vi "GetFusedHeading.vi"(11 "navX Device TypeDef":T1={"navX Interface Protocol"=enum."SPI", "navX Interface Protocol TypeDefs"={"SPIDevRef"={"DevStatus"={"status"=FALSE, "code"=0, "source"=""}, "Handle"=0, "SPI Bus"=enum."SPI On-Board, CS0"}, "I2CDevRef"={"DevStatus"={"status"=FALSE, "code"=0, "source"=""}, "Device Address"=0, "Handle"=0, "I2C Bus"=enum."Invalid"}}, "navX System Information"={"Board Information"={"WhoAmI (50 | 0x32)"=0, "Board Revision"=0, "Firmware Major Version"=0, "Firmware Minor Version"=0, "NAVX_BOARD_CAPABILITY"={"OMNIMOUNT"=FALSE, "YAW_RESET"=FALSE, "VEL_AND_DISP"=FALSE}, "NAVX_BOARD_YAW_AXIS"={"BOARD_YAW_AXIS_UP"=FALSE, "BOARD_YAW_AXIS"=0}}, "Status"={"Update Rate Hz"=0, "Accelerometer Full-Scale Range"=0, "Gyro Full-Scale Range"=0, "NAVX_OP_STATUS"=0, "NAVX_CAL_STATUS"=0, "NAVX_SELFTEST_STATUS"=0, "NAVX_SENSOR_STATUS"={"MOVING"=FALSE, "YAW_STABLE"=FALSE, "MAG_DISTURBANCE"=FALSE, "ALTITUDE_VALID"=FALSE, "SEALEVEL_PRESS_SET"=FALSE, "FUSED_HEADING_VALID"=FALSE}}, "Offsets"={"Yaw"=0.0, "Quat W"=0.0, "Quat X"=0.0, "Quat Y"=0.0, "Quat Z"=0.0}, "LastSampleTimestamp"=0.0, "LastSampleValid"=FALSE}, "navX Common Information"={"Update Rate (4Hz-60Hz)"=50, "refnum name"="", "error"={"status"=FALSE, "code"=0, "source"=""}, "LastSampleFPGATimestamp"=0.0}} {"navX Common Information"."Update Rate (4Hz-60Hz)" min=4 max=60 step=1; "navX System Information"."Status"."NAVX_OP_STATUS" items=["INITIALIZING", "SELFTEST_IN_PROGRESS", "ERROR", "IMU_AUTOCAL_IN_PROGRESS", "NORMAL"]; "navX System Information"."Status"."NAVX_CAL_STATUS" items=["IMU_CAL_STATE_MASK"=3, "IMU_CAL_INPROGRESS"=0, "IMU_CAL_ACCUMULATE"=1, "IMU_CAL_COMPLETE"=2, "MAG_CAL_COMPLETE"=4, "BARO_CAL_COMPLETE"=8]; "navX Interface Protocol TypeDefs"."I2CDevRef"."Device Address" format="%.0x"}) -> (1 "Valid?":bool, 2 "Fused Heading":dbl, 3 "navX Device TypeDef":T1={"navX Interface Protocol"=enum."SPI", "navX Interface Protocol TypeDefs"={"SPIDevRef"={"DevStatus"={"status"=FALSE, "code"=0, "source"=""}, "Handle"=0, "SPI Bus"=enum."SPI On-Board, CS0"}, "I2CDevRef"={"DevStatus"={"status"=FALSE, "code"=0, "source"=""}, "Device Address"=0, "Handle"=0, "I2C Bus"=enum."Invalid"}}, "navX System Information"={"Board Information"={"WhoAmI (50 | 0x32)"=0, "Board Revision"=0, "Firmware Major Version"=0, "Firmware Minor Version"=0, "NAVX_BOARD_CAPABILITY"={"OMNIMOUNT"=FALSE, "YAW_RESET"=FALSE, "VEL_AND_DISP"=FALSE}, "NAVX_BOARD_YAW_AXIS"={"BOARD_YAW_AXIS_UP"=FALSE, "BOARD_YAW_AXIS"=0}}, "Status"={"Update Rate Hz"=0, "Accelerometer Full-Scale Range"=0, "Gyro Full-Scale Range"=0, "NAVX_OP_STATUS"=0, "NAVX_CAL_STATUS"=0, "NAVX_SELFTEST_STATUS"=0, "NAVX_SENSOR_STATUS"={"MOVING"=FALSE, "YAW_STABLE"=FALSE, "MAG_DISTURBANCE"=FALSE, "ALTITUDE_VALID"=FALSE, "SEALEVEL_PRESS_SET"=FALSE, "FUSED_HEADING_VALID"=FALSE}}, "Offsets"={"Yaw"=0.0, "Quat W"=0.0, "Quat X"=0.0, "Quat Y"=0.0, "Quat Z"=0.0}, "LastSampleTimestamp"=0.0, "LastSampleValid"=FALSE}, "navX Common Information"={"Update Rate (4Hz-60Hz)"=50, "refnum name"="", "error"={"status"=FALSE, "code"=0, "source"=""}, "LastSampleFPGATimestamp"=0.0}} {"navX Common Information"."Update Rate (4Hz-60Hz)" min=4 max=60 step=1; "navX System Information"."Status"."NAVX_OP_STATUS" items=["INITIALIZING", "SELFTEST_IN_PROGRESS", "ERROR", "IMU_AUTOCAL_IN_PROGRESS", "NORMAL"]; "navX System Information"."Status"."NAVX_CAL_STATUS" items=["IMU_CAL_STATE_MASK"=3, "IMU_CAL_INPROGRESS"=0, "IMU_CAL_ACCUMULATE"=1, "IMU_CAL_COMPLETE"=2, "MAG_CAL_COMPLETE"=4, "BARO_CAL_COMPLETE"=8]; "navX Interface Protocol TypeDefs"."I2CDevRef"."Device Address" format="%.0x"})   [LabVIEW 2015, in "navX-MXP IMU.lvlib"]
doc: "This VI gets Fused Heading data from a navX MXP unit."
uses:
  navX-MXP IMU.lvlib
  TypeDefs/navX Device TypeDef.ctl
  TypeDefs/Value TypeDefs/navX Interface Protocol.ctl
  <vilib>/Rock Robotics/WPI/SPI/WPI_SPIDevRef.ctl
  <vilib>/Rock Robotics/SystemInterfaces/spilib/spi_bus.ctl
  <vilib>/Rock Robotics/WPI/I2C/WPI_I2CDevRef.ctl
  <vilib>/Rock Robotics/SystemInterfaces/i2clib/i2c_bus.ctl
  TypeDefs/Data TypeDefs/navX Board Information.ctl
  TypeDefs/Value TypeDefs/navX NAVX_BOARD_CAPABILITY.ctl
  TypeDefs/Value TypeDefs/navX NAVX_BOARD_YAW_AXIS.ctl
  TypeDefs/Data TypeDefs/navX Status Data.ctl
  TypeDefs/Value TypeDefs/navX NAVX_OP_STATUS.ctl
  TypeDefs/Value TypeDefs/navX NAVX_CAL_STATUS.ctl
  TypeDefs/Value TypeDefs/navX NAVX_SENSOR_STATUS.ctl
  TypeDefs/Data TypeDefs/navX Offsets Data.ctl
  TypeDefs/Value TypeDefs/navX Update Rate.ctl
  TypeDefs/Value TypeDefs/navX Device Registers.ctl
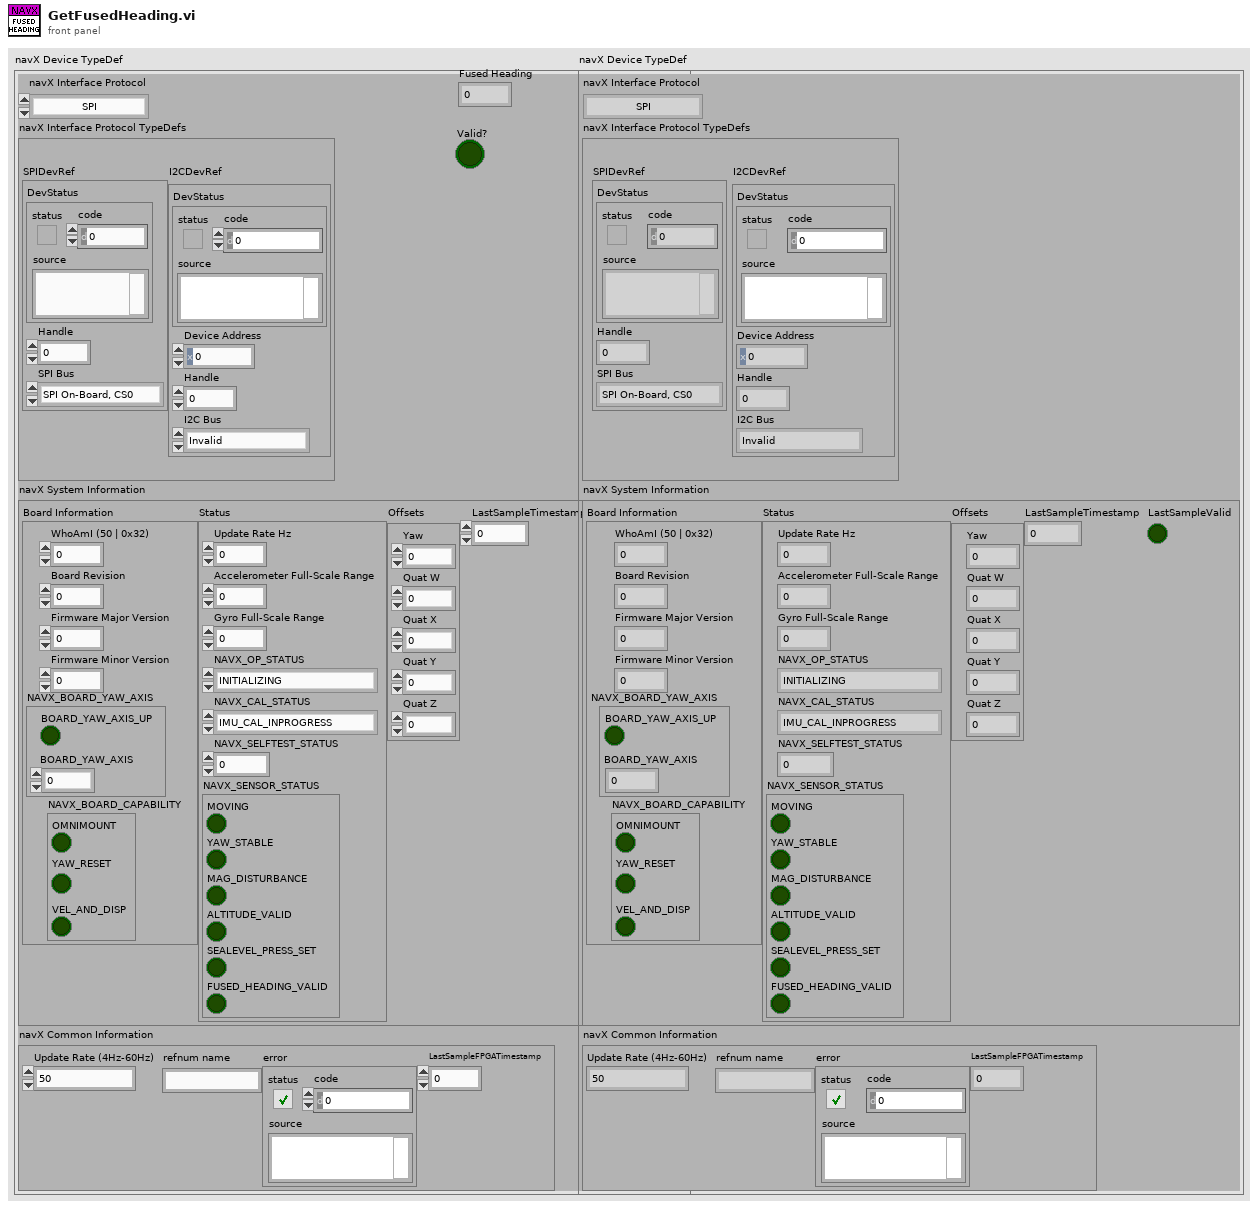
[diagram p1: front panel]
types:
  T1 = typedef "navX-MXP IMU.lvlib/navX Device TypeDef.ctl" = cluster{"navX Interface Protocol":T2, "navX Interface Protocol TypeDefs":cluster{"SPIDevRef":T3, "I2CDevRef":T5}, "navX System Information":cluster{"Board Information":T7, "Status":T10, "Offsets":T14, "LastSampleTimestamp":dbl, "LastSampleValid":bool}, "navX Common Information":cluster{"Update Rate (4Hz-60Hz)":T15, "refnum name":string, "error":errorcluster, "LastSampleFPGATimestamp":dbl}}
  T2 = typedef "navX-MXP IMU.lvlib/navX Interface Protocol.ctl" = enum16{"SPI", "I2C", "SERIAL"}
  T3 = typedef "WPI_SPIDevRef.ctl" = cluster{"DevStatus":errorcluster, "Handle":i32, "SPI Bus":T4}
  T4 = typedef "spi_bus.ctl" = enum16{"SPI On-Board, CS0", "SPI On-Board, CS1", "SPI On-Board, CS2", "SPI On-Board, CS3", "SPI MXP", "Invalid"}
  T5 = typedef "WPI_I2CDevRef.ctl" = cluster{"DevStatus":errorcluster, "Device Address":u8, "Handle":i32, "I2C Bus":T6}
  T6 = typedef "i2c_bus.ctl" = enum16{"I2C On-Board", "I2C MXP", "Invalid"}
  T7 = typedef "navX-MXP IMU.lvlib/navX Board Information.ctl" = cluster{"WhoAmI (50 | 0x32)":u8, "Board Revision":u8, "Firmware Major Version":u8, "Firmware Minor Version":u8, "NAVX_BOARD_CAPABILITY":T8, "NAVX_BOARD_YAW_AXIS":T9}
  T8 = typedef "navX-MXP IMU.lvlib/navX NAVX_BOARD_CAPABILITY.ctl" = cluster{"OMNIMOUNT":bool, "YAW_RESET":bool, "VEL_AND_DISP":bool}
  T9 = typedef "navX-MXP IMU.lvlib/navX NAVX_BOARD_YAW_AXIS.ctl" = cluster{"BOARD_YAW_AXIS_UP":bool, "BOARD_YAW_AXIS":u8}
  T10 = typedef "navX-MXP IMU.lvlib/navX Status Data.ctl" = cluster{"Update Rate Hz":u8, "Accelerometer Full-Scale Range":u8, "Gyro Full-Scale Range":u16, "NAVX_OP_STATUS":T11, "NAVX_CAL_STATUS":T12, "NAVX_SELFTEST_STATUS":u8, "NAVX_SENSOR_STATUS":T13}
  T11 = typedef "navX-MXP IMU.lvlib/navX NAVX_OP_STATUS.ctl" = u8
  T12 = typedef "navX-MXP IMU.lvlib/navX NAVX_CAL_STATUS.ctl" = u8
  T13 = typedef "navX-MXP IMU.lvlib/navX NAVX_SENSOR_STATUS.ctl" = cluster{"MOVING":bool, "YAW_STABLE":bool, "MAG_DISTURBANCE":bool, "ALTITUDE_VALID":bool, "SEALEVEL_PRESS_SET":bool, "FUSED_HEADING_VALID":bool}
  T14 = typedef "navX-MXP IMU.lvlib/navX Offsets Data.ctl" = cluster{"Yaw":dbl, "Quat W":dbl, "Quat X":dbl, "Quat Y":dbl, "Quat Z":dbl}
  T15 = typedef "navX-MXP IMU.lvlib/navX Update Rate.ctl" = u8
  T16 = typedef "navX-MXP IMU.lvlib/navX Device Registers.ctl" = u8
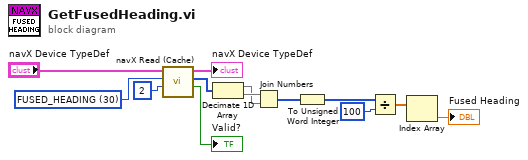
[diagram p0: block diagram]
diagram:
  w11 = T16 30 items=["WHOAMI"=0, "HW_REV"=1, "FW_VER_MAJOR"=2, "FW_VER_MINOR"=3, "UPDATE_RATE_HZ"=4, "ACCEL_FSR_G"=5, "GYRO_FSR_DPS"=6, "OP_STATUS"=8, "CAL_STATUS"=9, "SELFTEST_STATUS"=10, "SENSOR_STATUS"=16, "TIMESTAMP"=18, "YAW"=22, "PITCH"=24, "ROLL"=26, "HEADING"=28, "FUSED_HEADING"=30, "ALTITUDE_I"=32, "ALTITUDE_D"=34, "LINERA_ACC_X"=36, "LINERA_ACC_Y"=38, "LINERA_ACC_Z"=40, "QUAT_W"=42, "QUAT_X"=44, "QUAT_Y"=46, "QUAT_Z"=48, "MPU_TEMP_C"=50, "GYRO_X"=52, "GYRO_Y"=54, "GYRO_Z"=56, "ACC_X"=58, "ACC_Y"=60, "ACC_Z"=62, "MAG_X"=64, "MAG_Y"=66, "MAG_Z"=68, "PRESSURE_I"=70, "PRESSURE_D"=72, "PRESSURE_TEMP"=74, "YAW_OFFSET"=76, "QUAT_OFFSET_W"=78, "QUAT_OFFSET_X"=80, "QUAT_OFFSET_Y"=82, "QUAT_OFFSET_Z"=84] ("Device Register")
  n1 = call "navX Read (Cache).vi"("Read Size (2)"=u8 2, "Device Register (WHOAMI)"=w11, "navX Device TypeDef"="navX Device TypeDef") -> ("Valid?"=→"Valid?":bool, "navX Data"=w4:u8[], "navX Device TypeDef"=→"navX Device TypeDef":T1)  [unwired: 6 in]
  n2 = Decimate 1D Array(w4) -> (w8:u8[], w9:u8[])
  n3 = Join Numbers(hi=w9, lo=w8) -> ((hi.lo)=w7:u16[])
  n4 = To Unsigned Word Integer(number=w7) -> (unsigned 16bit integer=w6:u16[])
  n5 = Divide(x=w6, y=100) -> (x/y=w3:dbl[])
  n6 = Index Array(array=w3) -> (element=→"Fused Heading":dbl)  [unwired: 1 in]
